vi "Set Stage Speed.vi"(8 "error in (no error)":errorcluster, 9 "Y Axis":u16, 10 "X Axis":u16, 11 "2-Axis Stage in":refnum<class "XY Stage Process.lvclass">) -> (0 "error out":errorcluster, 3 "2-Axis Stage out":refnum<class "XY Stage Process.lvclass">)   [LabVIEW 2022 SP3, in "XY Stage Process.lvlib" / "XY Stage Process.lvclass"]
uses:
  XY Stage Process.lvclass
  XY Stage Process.lvclass/XY Stage Process.ctl
  Axis Objects/iMotion Controller/iMotion Controller.lvclass
  Process State Data/Process State Data.lvclass
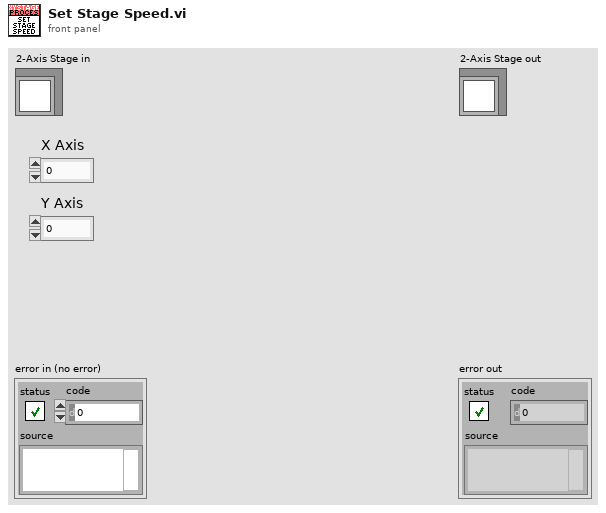
[diagram p1: front panel]
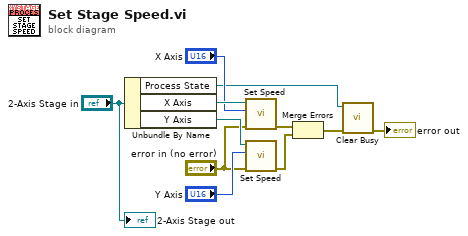
[diagram p0: block diagram]
diagram:
  n1 = Unbundle By Name("2-Axis Stage in") -> ("Process State"=w2:refnum<data-value>, "X Axis"=w10:refnum<class "iMotion Controller.lvclass">, "Y Axis"=w7:refnum<class "iMotion Controller.lvclass">)
  n2 = call-dynamic "Set Speed.vi"("error in (no error)"="error in (no error)", "Speed"="X Axis", "iMotion Controller in"=w10) -> ("error out"=w5:errorcluster)  [unwired: 7 in, 1 out]
  n3 = call-dynamic "Set Speed.vi"("error in (no error)"="error in (no error)", "Speed"="Y Axis", "iMotion Controller in"=w7) -> ("error out"=w4:errorcluster)  [unwired: 7 in, 1 out]
  n4 = Merge Errors(w5, w4) -> (w3:errorcluster)
  n5 = call "Clear Busy.vi"("error in (no error)"=w3, "Process State"=w2) -> ("error out"=→"error out":errorcluster)  [unwired: 8 in, 1 out]
  "2-Axis Stage out" <- "2-Axis Stage in"
